vi "Offset Table Headers.vi"(6 "Rigid Connection":bool=TRUE, 7 "Coordinate Space":bool caption="Coord", 9 "Number of\nLBCBs":T1=enum."2", 11 "Offset Type":T2=enum."Forces") -> (0 "Visible":bool[](array[boolean]), 1 "Column DOF Headers":string[](array[string])=["LBCB 1 Offset", "LBCB 1 Current", "LBCB 2 Offset", "LBCB 2 Current", "Comb Offset", "Comb Current"], 2 "Column LBCB Headers":string[](array[string])=["LBCB 1 Offset", "LBCB 1 Current", "LBCB 2 Offset", "LBCB 2 Current", "Comb Offset", "Comb Current"], 3 "Row Headers":string[](array[string])=["", "Fx (lbs)", "Fy (lbs)", "Fz (lbs)", "Mx(lb*inches)", "My(lb*inches)", "Mz(lb*inches)"], 4 "Ext Visible":bool)   [LabVIEW 2013]
uses:
  lib/Offsets/Offset Types.ctl
  lib/Data Access Objects/Application/Number Of LBCBs.ctl
  lib/Apps/Unit Label Type.ctl
  lib/Data Access Objects/Metadata/Persistant DAO Actions.ctl
panel:
  in  "LBCB Names":string[](array[string])=["LBCB 1", "LBCB 2", "Comb"]
  in  "Row Header\nChannel Type":string[](array[string])=["Command", "Reading"]
  in  "Cartesian\nForce":string[](array[string])=["Fx", "Fy", "Fz", "Mx", "My", "Mz"]
  in  "Cartesian\nDisp":string[](array[string])=["Dx", "Dy", "Dz", "Rx", "Ry", "Rz"]
  in  "Actuators":string[](array[string])=["X1", "X2", "Y1", "Z1", "Z2", "Z3"]
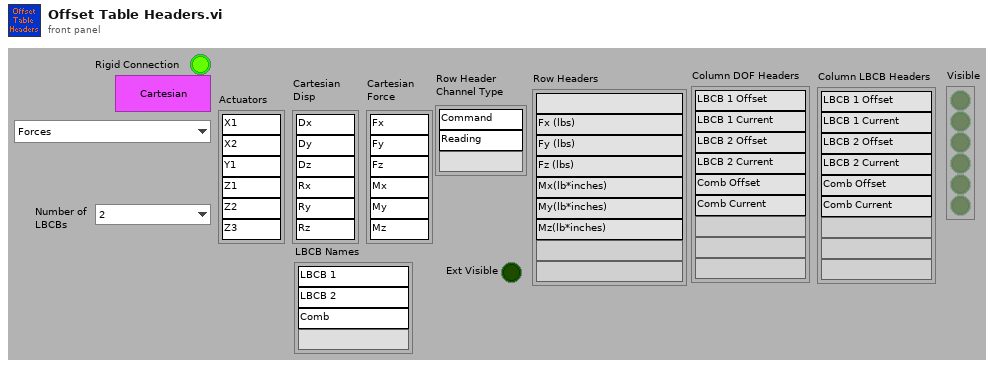
[diagram p1: front panel]
types:
  T1 = typedef "Number Of LBCBs.ctl" = enum16{"1", "2"}
  T2 = typedef "Offset Types.ctl" = enum16{"Displacements", "Forces", "External Sensors"}
  T3 = typedef "Unit Label Type.ctl" = enum16{"Actuator Displacement", "Actuator Force", "Cartesian Force", "Cartesian Translation", "Cartesian Rotation", "Cartesian Moment"}
  T4 = typedef "Persistant DAO Actions.ctl" = enum16{"Init", "Get", "Set", "Load", "Save"}
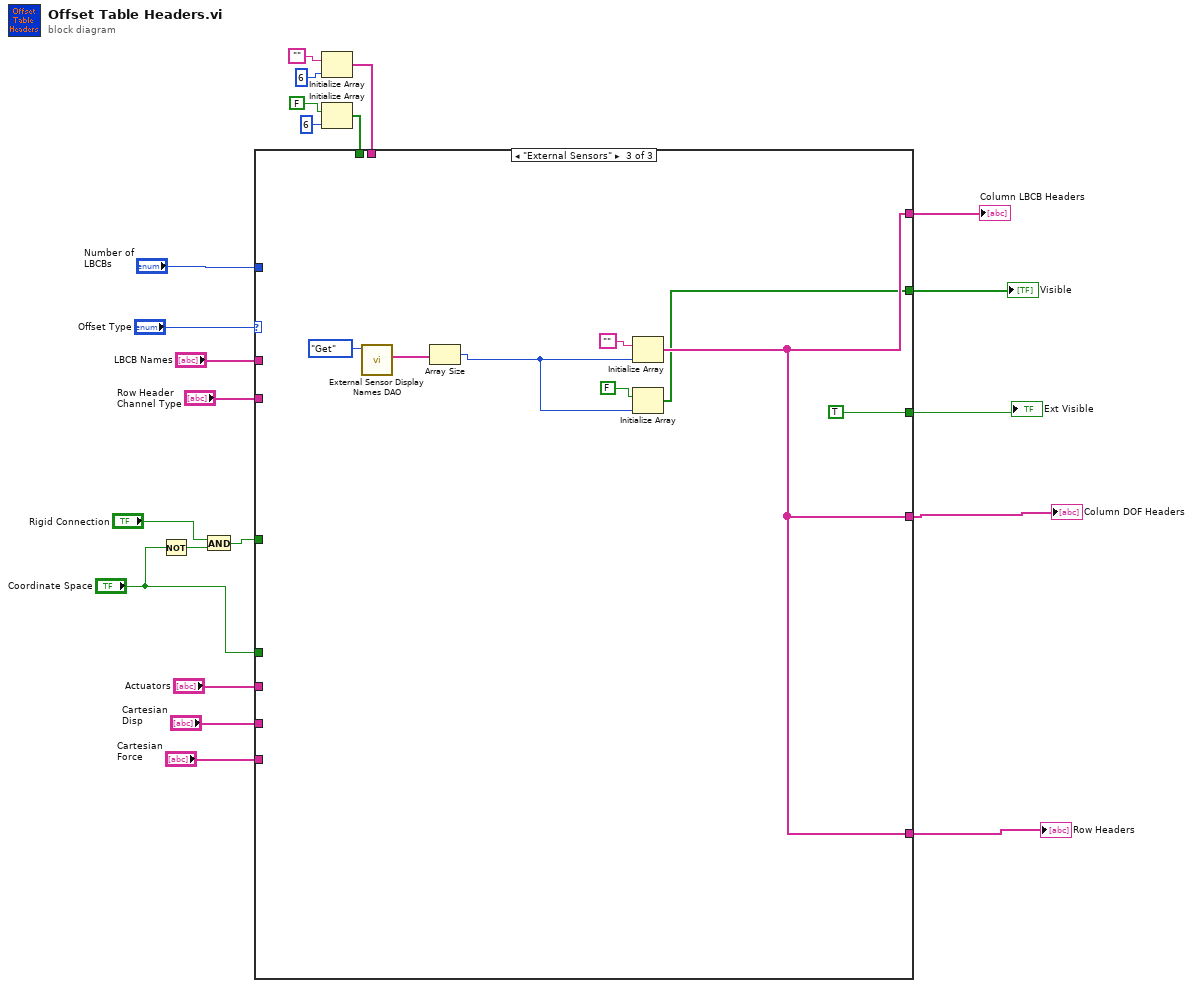
[diagram p0: block diagram]
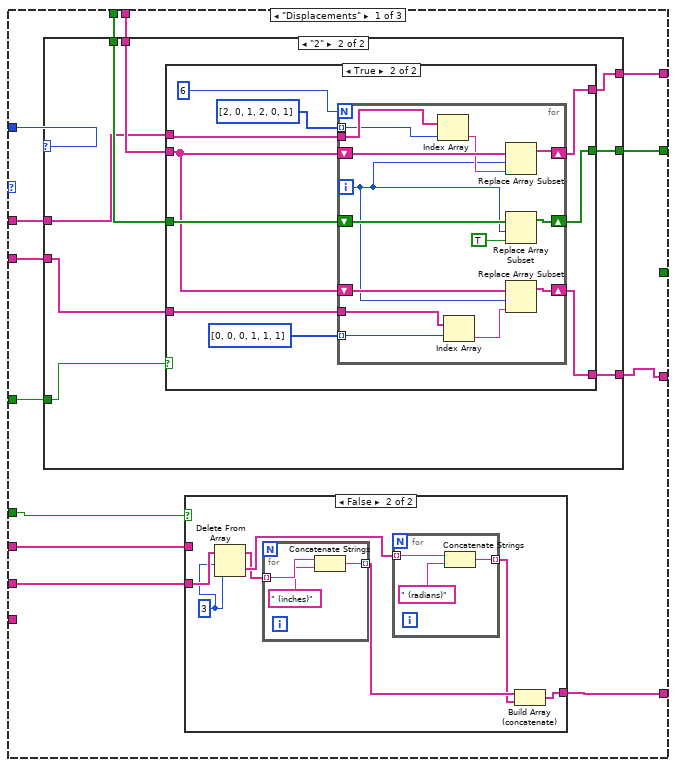
[diagram p2: hidden frame]
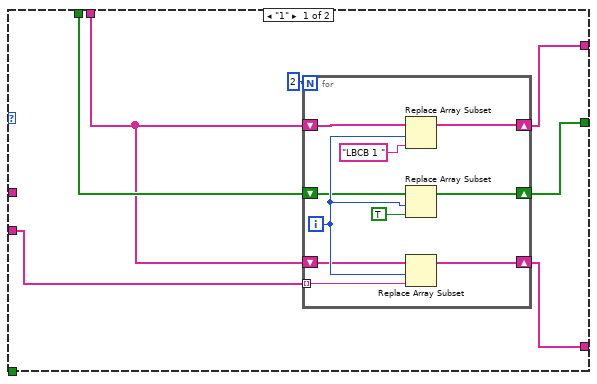
[diagram p3: hidden frame]
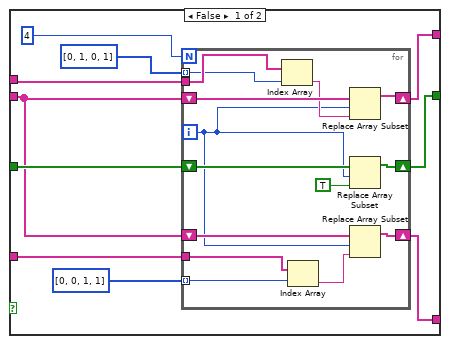
[diagram p4: hidden frame]
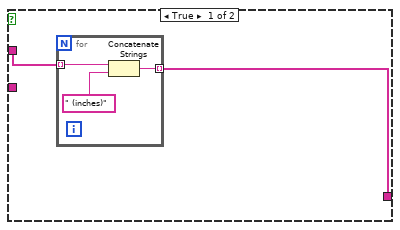
[diagram p5: hidden frame]
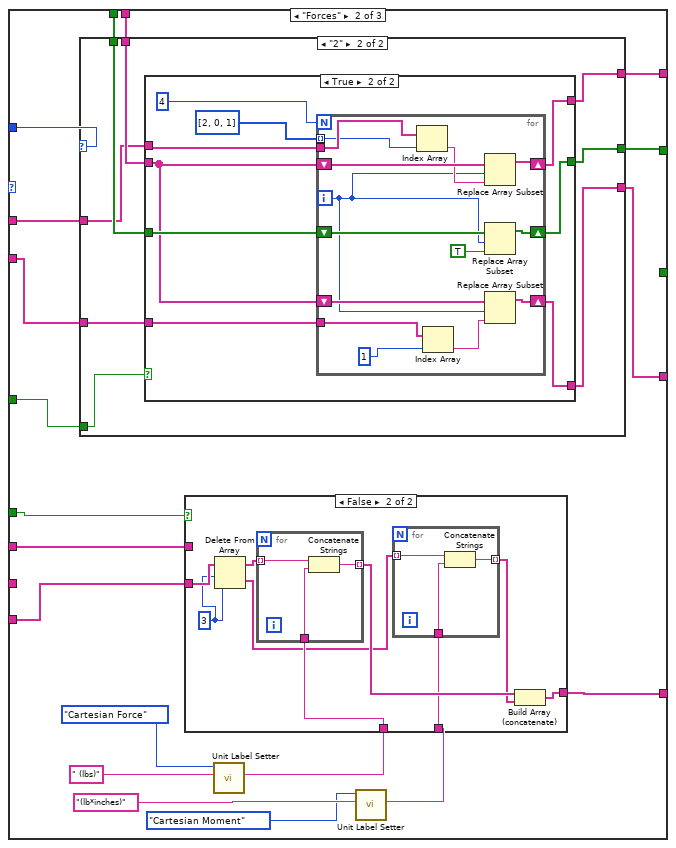
[diagram p6: hidden frame]
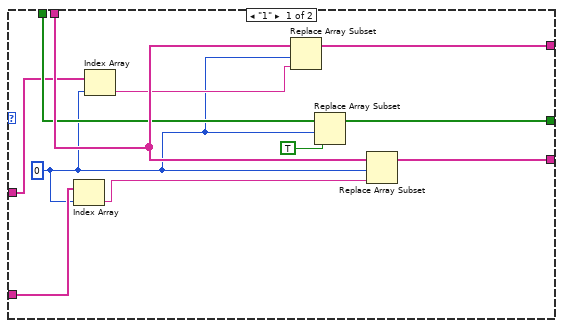
[diagram p7: hidden frame]
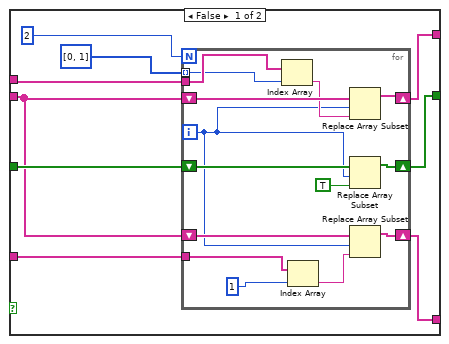
[diagram p8: hidden frame]
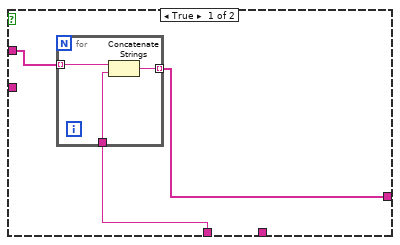
[diagram p9: hidden frame]
diagram:
  n1 = Not(x="Coordinate Space") -> (.not. x?=w12:bool)
  n2 = And(x="Rigid Connection", y=w12) -> (x .and. y?=w14:bool)
  n3 = Initialize Array("", 6 ("dimension size")) -> (w5:string[])
  n4 = Initialize Array(FALSE, 6 ("dimension size")) -> (w4:bool[])
  n5 = case shown="\"External Sensors\"" "Offset Type" {
    tunnel: [w33 w143 w233] -> w15
    tunnel: [w24 w139 w233] -> w3
    tunnel: "Coordinate Space" -> [w35 w145 _]
    tunnel: "Actuators" -> [w34 w144 _]
    tunnel: "Number of\nLBCBs" -> [w32 w142 _]
    tunnel: "Cartesian\nDisp" -> [w31 _ _]
    tunnel: "Cartesian\nForce" -> [_ w141 _]
    tunnel: w14 -> [w30 w140 _]
    tunnel: "Row Header\nChannel Type" -> [w29 w133 _]
    tunnel: [w28 w137 w233] -> w11
    tunnel: [w27 w135 w232] -> w10
    tunnel: w5 -> [w26 w138 _]
    tunnel: w4 -> [w25 w136 _]
    tunnel: "LBCB Names" -> [w23 w134 _]
    tunnel: [_ _ TRUE] -> w1
    frame "Displacements" {
      n6 = case shown="\"2\"" w32 {
        tunnel: [w37 w56] -> w24
        tunnel: w30 -> [_ w54]
        tunnel: w29 -> [w40 w59]
        tunnel: [w41 w60] -> w28
        tunnel: [w36 w55] -> w27
        tunnel: w26 -> [w38 w57]
        tunnel: w25 -> [w39 w58]
        tunnel: w23 -> [_ w53]
        frame "1" {
          n7 = for {
            N: 2 -> [_]
            shift-right: [w50] -> w41
            shift-left: w38 -> [w52]
            tunnel: w40 -> [w48] mode=indexing
            shift-right: [w46] -> w36
            shift-left: w39 -> [w47]
            shift-right: [w44] -> w37
            shift-left: w38 -> [w43]
            i -> [w49]
            n8 = Replace Array Subset(array=w52, new element="LBCB 1 " ("string"), index=w49) -> (w50:string[])
            n9 = Replace Array Subset(array=w47, new element=TRUE ("new element/subarray"), index=w49) -> (w46:bool[])
            n10 = Replace Array Subset(array=w43, new element=w48, index=w49) -> (w44:string[])
          }
        }
        frame "2" {
          n11 = case shown="True" w54 {
            tunnel: [w70 w94] -> w60
            tunnel: w59 -> [w69 w93]
            tunnel: w58 -> [w68 w92]
            tunnel: w57 -> [w67 w91]
            tunnel: [w66 w90] -> w56
            tunnel: [w65 w89] -> w55
            tunnel: w53 -> [w63 w87]
            frame False {
              n12 = for {
                N: 4 -> [_]
                shift-right: [w83] -> w70
                shift-left: w67 -> [w84]
                tunnel: w69 -> [w75]
                shift-right: [w81] -> w65
                shift-left: w68 -> [w82]
                shift-right: [w79] -> w66
                shift-left: w67 -> [w78]
                tunnel: w63 -> [w77]
                tunnel: i32[] [0, 1, 0, 1] -> [w73] mode=indexing
                tunnel: i32[] [0, 0, 1, 1] -> [w71] mode=indexing
                i -> [w72]
                n13 = Index Array(array=w77, index=w73) -> (element=w76:string)
                n14 = Index Array(array=w75, index=w71) -> (element=w74:string)
                n15 = Replace Array Subset(array=w84, new element=w76, index=w72) -> (w83:string[])
                n16 = Replace Array Subset(array=w82, new element=TRUE ("new element/subarray"), index=w72) -> (w81:bool[])
                n17 = Replace Array Subset(array=w78, new element=w74, index=w72) -> (w79:string[])
              }
            }
            frame True {
              n18 = for {
                N: 6 -> [_]
                shift-right: [w107] -> w94
                shift-left: w91 -> [w108]
                tunnel: w93 -> [w99]
                shift-right: [w105] -> w89
                shift-left: w92 -> [w106]
                shift-right: [w103] -> w90
                shift-left: w91 -> [w102]
                tunnel: w87 -> [w101]
                tunnel: i32[] [2, 0, 1, 2, 0, 1] -> [w97] mode=indexing
                tunnel: i32[] [0, 0, 0, 1, 1, 1] -> [w95] mode=indexing
                i -> [w96]
                n19 = Index Array(array=w101, index=w97) -> (element=w100:string)
                n20 = Index Array(array=w99, index=w95) -> (element=w98:string)
                n21 = Replace Array Subset(array=w108, new element=w100, index=w96) -> (w107:string[])
                n22 = Replace Array Subset(array=w106, new element=TRUE ("new element/subarray"), index=w96) -> (w105:bool[])
                n23 = Replace Array Subset(array=w102, new element=w98, index=w96) -> (w103:string[])
              }
            }
          }
        }
      }
      n24 = case shown="False" w35 {
        tunnel: w34 -> [w110 _]
        tunnel: [w109 w118] -> w33
        tunnel: w31 -> [_ w117]
        frame True {
          n25 = for {
            tunnel: w110 -> [w113] mode=indexing
            tunnel: [w111] -> w109 mode=indexing
            n26 = Concatenate Strings(w113, " (inches)") -> (w111:string)
          }
        }
        frame False {
          w116 = 3 ("index")
          n27 = Delete From Array(array=w117, length=w116, index=w116) -> (deleted portion=w115:string[], array with subset deleted=w114:string[])
          n28 = for {
            tunnel: w114 -> [w126] mode=indexing
            tunnel: [w124] -> w120 mode=indexing
            n29 = Concatenate Strings(w126, " (inches)") -> (w124:string)
          }
          n30 = for {
            tunnel: w115 -> [w123] mode=indexing
            tunnel: [w121] -> w119 mode=indexing
            n31 = Concatenate Strings(w123, " (radians)") -> (w121:string)
          }
          n32 = Build Array (concatenate)(w120, w119) -> (w118:string[])
        }
      }
    }
    frame "Forces" {
      n33 = case shown="\"2\"" w142 {
        tunnel: [w149 w160] -> w139
        tunnel: w140 -> [_ w164]
        tunnel: w138 -> [w156 w159]
        tunnel: [w152 w163] -> w137
        tunnel: [w154 w161] -> w135
        tunnel: w136 -> [w155 w162]
        tunnel: w134 -> [w151 w158]
        tunnel: w133 -> [w148 w157]
        frame "1" {
          w147 = 0 ("index")
          n34 = Index Array(array=w148, index=w147) -> (element=w146:string)
          n35 = Index Array(array=w151, index=w147) -> (element=w150:string)
          n36 = Replace Array Subset(array=w156, new element=w150, index=w147) -> (w152:string[])
          n37 = Replace Array Subset(array=w155, new element=TRUE ("new element/subarray"), index=w147) -> (w154:bool[])
          n38 = Replace Array Subset(array=w156, new element=w146, index=w147) -> (w149:string[])
        }
        frame "2" {
          n39 = case shown="True" w164 {
            tunnel: [w173 w196] -> w163
            tunnel: w157 -> [w172 w195]
            tunnel: w162 -> [w171 w194]
            tunnel: w159 -> [w170 w193]
            tunnel: [w169 w192] -> w160
            tunnel: [w168 w191] -> w161
            tunnel: w158 -> [w166 w189]
            frame False {
              n40 = for {
                N: 2 -> [_]
                shift-right: [w186] -> w173
                shift-left: w170 -> [w187]
                tunnel: w172 -> [w178]
                shift-right: [w184] -> w168
                shift-left: w171 -> [w185]
                shift-right: [w182] -> w169
                shift-left: w170 -> [w181]
                tunnel: w166 -> [w180]
                tunnel: i32[] [0, 1] -> [w176] mode=indexing
                i -> [w175]
                n41 = Index Array(array=w180, index=w176) -> (element=w179:string)
                n42 = Index Array(array=w178, index=1) -> (element=w177:string)
                n43 = Replace Array Subset(array=w187, new element=w179, index=w175) -> (w186:string[])
                n44 = Replace Array Subset(array=w185, new element=TRUE ("new element/subarray"), index=w175) -> (w184:bool[])
                n45 = Replace Array Subset(array=w181, new element=w177, index=w175) -> (w182:string[])
              }
            }
            frame True {
              n46 = for {
                N: 4 -> [_]
                shift-right: [w209] -> w196
                shift-left: w193 -> [w210]
                tunnel: w195 -> [w201]
                shift-right: [w207] -> w191
                shift-left: w194 -> [w208]
                shift-right: [w205] -> w192
                shift-left: w193 -> [w204]
                tunnel: w189 -> [w203]
                tunnel: i32[] [2, 0, 1] -> [w199] mode=indexing
                i -> [w198]
                n47 = Index Array(array=w203, index=w199) -> (element=w202:string)
                n48 = Index Array(array=w201, index=1) -> (element=w200:string)
                n49 = Replace Array Subset(array=w210, new element=w202, index=w198) -> (w209:string[])
                n50 = Replace Array Subset(array=w208, new element=TRUE ("new element/subarray"), index=w198) -> (w207:bool[])
                n51 = Replace Array Subset(array=w204, new element=w200, index=w198) -> (w205:string[])
              }
            }
          }
        }
      }
      n52 = call "Unit Label Setter.vi"("Input String"=" (lbs)", "Label Type"=Unit_Label_Type."Cartesian Force") -> ("Output String"=w130:string)  [unwired: 9 in]
      n53 = call "Unit Label Setter.vi"("Input String"="(lb*inches)", "Label Type"=Unit_Label_Type."Cartesian Moment") -> ("Output String"=w127:string)  [unwired: 9 in]
      n54 = case shown="False" w145 {
        tunnel: w144 -> [w213 _]
        tunnel: [w212 w223] -> w143
        tunnel: w141 -> [_ w220]
        tunnel: w130 -> [w211 w222]
        tunnel: w127 -> [_ w221]
        frame True {
          n55 = for {
            tunnel: w213 -> [w216] mode=indexing
            tunnel: [w215] -> w212 mode=indexing
            tunnel: w211 -> [w214]
            n56 = Concatenate Strings(w216, w214) -> (w215:string)
          }
        }
        frame False {
          w217 = 3 ("index")
          n57 = Delete From Array(array=w220, length=w217, index=w217) -> (deleted portion=w218:string[], array with subset deleted=w219:string[])
          n58 = for {
            tunnel: w219 -> [w231] mode=indexing
            tunnel: [w230] -> w225 mode=indexing
            tunnel: w222 -> [w229]
            n59 = Concatenate Strings(w231, w229) -> (w230:string)
          }
          n60 = for {
            tunnel: w218 -> [w228] mode=indexing
            tunnel: [w227] -> w224 mode=indexing
            tunnel: w221 -> [w226]
            n61 = Concatenate Strings(w228, w226) -> (w227:string)
          }
          n62 = Build Array (concatenate)(w225, w224) -> (w223:string[])
        }
      }
    }
    frame "External Sensors" {
      n63 = call "External Sensor Display Names DAO.vi"("Persistent DAO Actions"=Persistant_DAO_Actions."Get") -> ("Display Name Out"=w235:string[])  [unwired: 8 in, 2 out]
      n64 = Array Size(array=w235) -> (size(s)=w234:i32)
      n65 = Initialize Array("", w234) -> (w233:string[])
      n66 = Initialize Array(FALSE, w234) -> (w232:bool[])
    }
  }
  "Row Headers" <- w15
  "Column DOF Headers" <- w3
  "Column LBCB Headers" <- w11
  "Visible" <- w10
  "Ext Visible" <- w1
